vi "Weather Station UI.vi"(10 "Lower Limit":dbl=10.0, 11 "Upper Limit":dbl=30.0) -> (1 "Warning":string, 2 "Temperature History":dbl(graph))   [LabVIEW 2010]
doc: "This is the main VI in the Weather Station Project. It contains the user interface for a temperature warning system. \n\nUser inputs: Maximum Temperature, Minimum Temperature, Temperature Units.\nOutputs: Current Temperature, Warning State"
uses:
  Supporting Files/Weather Station States.ctl
panel:
  in  "Weather Data":dynamicdata(graph)
  in  "stop":bool
  in  "Wind Upper Limit":dbl(slide)=50.0 scale=0.0..100.0
  out "Wind Speed History":dbl(graph)
  # "Celcius"
  # "Temperature Ranges"
  # "Heat \nStroke"
  # "Freeze"
  # "kph"
  # "Maximum Safe Wind Speed"
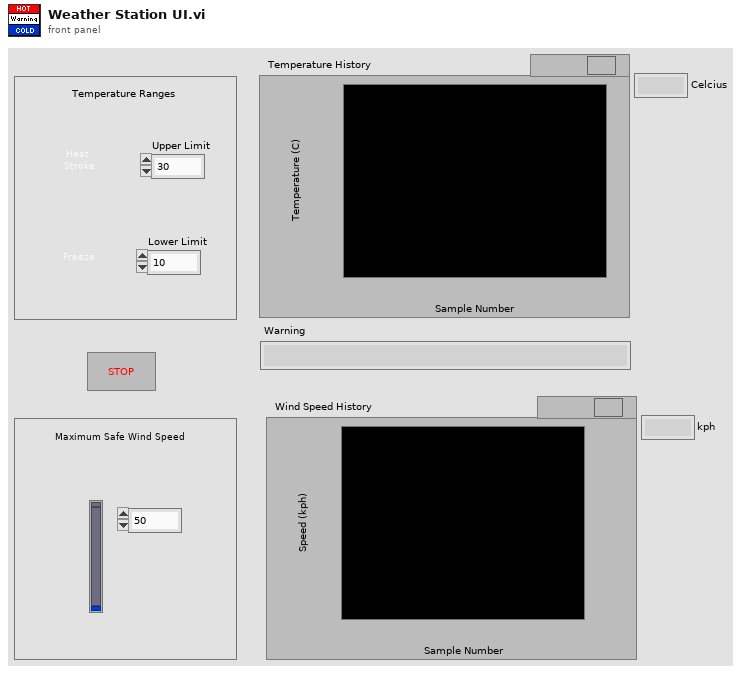
[diagram p1: front panel]
types:
  T1 = cluster{"Temperature":dbl, "T Upper Limit":dbl, "T Lower Limit":dbl, "Wind Speed":dbl, "Wind Upper Limit":dbl, "Warning":string, "Time":dbl}
  T2 = typedef "Weather Station States.ctl" = enum16{"Analysis", "Process UI", "Set Warning", "Data Log", "Stop"}
  T3 = enum32{"invalid app kind", "Development System", "Run Time System", "Student Edition", "Embedded LabVIEW", "Evaluation", "Custom"}
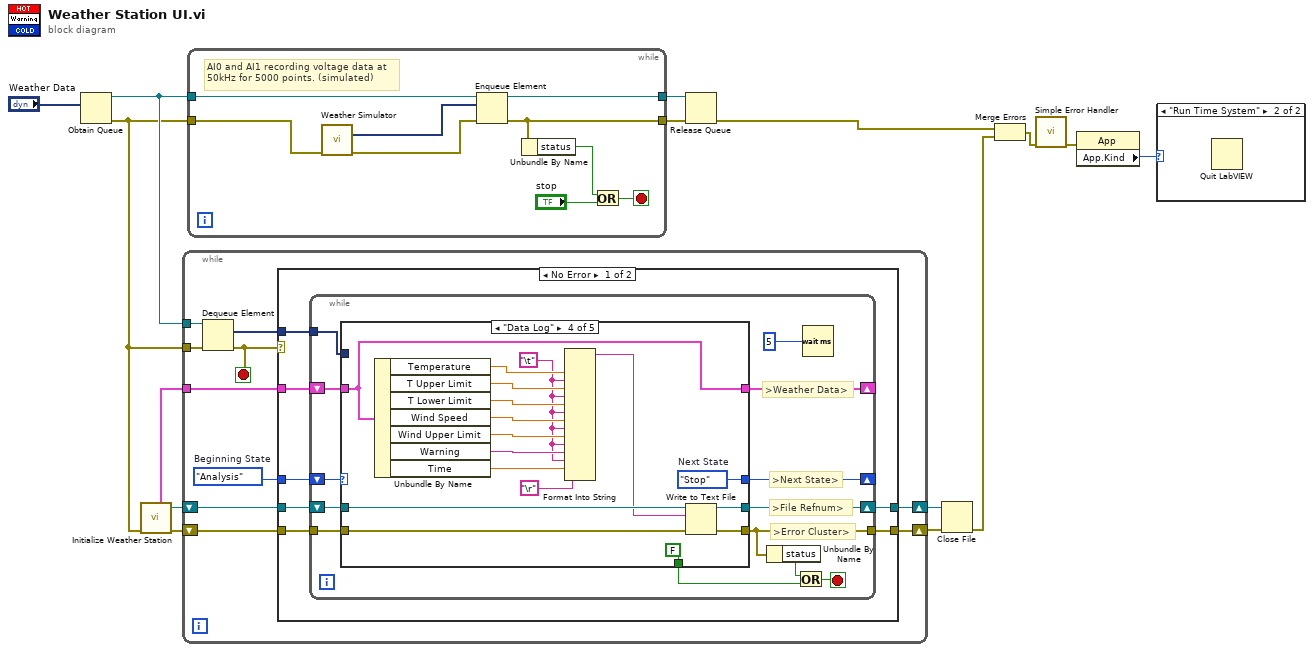
[diagram p0: block diagram]
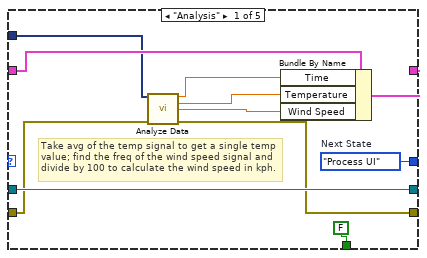
[diagram p3: hidden frame]
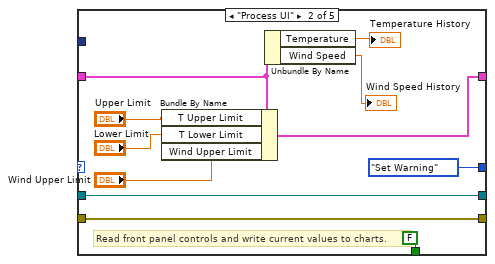
[diagram p4: hidden frame]
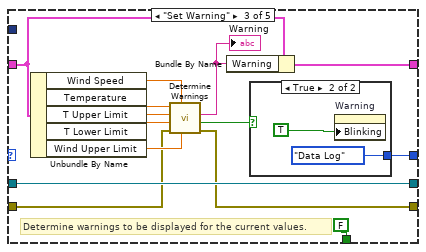
[diagram p5: hidden frame]
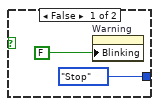
[diagram p6: hidden frame]
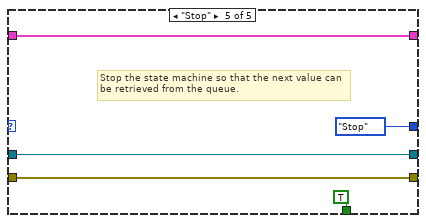
[diagram p7: hidden frame]
diagram:
  n1 = Obtain Queue(element data type="Weather Data") -> (queue out=w12:refnum<queue>, error out=w3:errorcluster)  [unwired: 4 in, 1 out]
  n2 = call "Initialize Weather Station.vi"("error in (no error)"=w3) -> ("error out"=w4:errorcluster, "file refnum"=w5:refnum<file>, "Weather Data"=w15:T1)  [unwired: 8 in]
  n3 = while {
    tunnel: w15 -> [w24]
    tunnel: w12 -> [w23]
    tunnel: w3 -> [w22]
    shift-right: [w25] -> w8
    shift-left: w5 -> [w21]
    shift-right: [w17] -> w7
    shift-left: w4 -> [w18]
    stop <- w20 stop-if-true
    w16 = Weather_Station_States."Analysis"  # Beginning State
    n4 = Dequeue Element(queue=w23, error in (no error)=w22) -> (element=w19:dynamicdata, error out=w20:errorcluster)  [unwired: 1 in, 2 out]
    n5 = case shown="No Error" w20 {
      tunnel: [w32 w108] -> w25
      tunnel: w24 -> [w31 _]
      tunnel: w21 -> [w30 w108]
      tunnel: w19 -> [w29 _]
      tunnel: w18 -> [w27 w109]
      tunnel: [w28 w109] -> w17
      tunnel: w16 -> [w26 _]
      frame No Error {
        n6 = while {
          shift-right: [w45] -> _
          shift-left: w26 -> [w37]
          shift-right: [w34] -> w32
          shift-left: w30 -> [w44]
          shift-right: [w38] -> _
          shift-left: w31 -> [w41]
          tunnel: w29 -> [w36]
          tunnel: [w35] -> w28
          tunnel: w27 -> [w33]
          stop <- w43 stop-if-true
          # ">Error Cluster>"
          # ">Weather Data>"
          # ">File Refnum>"
          # ">Next State>"
          n7 = case shown="\"Data Log\"" w37 {
            tunnel: [w56 Weather_Station_States."Set Warning" ("Next State") w80 w102 Weather_Station_States."Stop" ("Next State")] -> w45
            tunnel: [w46 w58 w70 w99 w103] -> w35
            tunnel: w44 -> [w52 w57 w77 w98 w104]
            tunnel: [w53 w67 w78 w96 w105] -> w38
            tunnel: w41 -> [w54 w64 w79 w96 w105]
            tunnel: [FALSE ("stop") FALSE ("stop") FALSE ("stop") FALSE ("stop") TRUE ("stop")] -> w40
            tunnel: w36 -> [w51 _ _ _ _]
            tunnel: [w52 w57 w77 w100 w104] -> w34
            tunnel: w33 -> [w50 w58 w71 w86 w103]
            frame "Analysis" {
              w56 = Weather_Station_States."Process UI"  # Next State
              # "Take avg of the temp signal to get a single temp value; find the freq of the wind speed signal and divide by 100 to calculate the wind speed in kph."
              n8 = call "Analyze Data.vi"("Weather Data"=w51, "error in"=w50) -> ("Time"=w49:dbl, "Temperature"=w48:dbl, "Wind Speed"=w47:dbl, "error out"=w46:errorcluster)  [unwired: 10 in]
              n9 = Bundle By Name(cluster=w54, "Time"=w49, "Temperature"=w48, "Wind Speed"=w47) -> (w53:T1)
            }
            frame "Process UI" {
              # "Read front panel controls and write current values to charts."
              n10 = Bundle By Name(cluster=w64, "T Upper Limit"="Upper Limit", "T Lower Limit"="Lower Limit", "Wind Upper Limit"="Wind Upper Limit") -> (w67:T1)
              n11 = Unbundle By Name(w64) -> ("Temperature"=→"Temperature History":dbl, "Wind Speed"=→"Wind Speed History":dbl)
            }
            frame "Set Warning" {
              # "Determine warnings to be displayed for the current values."
              n12 = Unbundle By Name(w79) -> ("Wind Speed"=w76:dbl, "Temperature"=w75:dbl, "T Upper Limit"=w74:dbl, "T Lower Limit"=w73:dbl, "Wind Upper Limit"=w72:dbl)
              n13 = call "Determine Warnings.vi"("Max Wind Speed"=w72, "Current Wind Speed"=w76, "error in (no error)"=w71, "Min Temp"=w73, "Max Temp"=w74, "Current Temp"=w75) -> ("error out"=w70:errorcluster, "Warning?"=w69:bool, "Warning Text"=w68:string)  [unwired: 3 in]
              "Warning" <- w68
              n14 = Bundle By Name(cluster=w79, "Warning"=w68) -> (w78:T1)
              n15 = case shown="True" w69 {
                tunnel: [Weather_Station_States."Stop" ("Next State") Weather_Station_States."Data Log" ("Next State")] -> w80
                frame False {
                  n16 = property on="Warning" class="Str"("Blinking"=FALSE) -> ()  [unwired: 2 in, 2 out]
                }
                frame True {
                  n17 = property on="Warning" class="Str"("Blinking"=TRUE) -> ()  [unwired: 2 in, 2 out]
                }
              }
            }
            frame "Data Log" {
              w88 = "\t"
              w102 = Weather_Station_States."Stop"  # Next State
              n18 = Unbundle By Name(w96) -> ("Temperature"=w95:dbl, "T Upper Limit"=w94:dbl, "T Lower Limit"=w93:dbl, "Wind Speed"=w92:dbl, "Wind Upper Limit"=w91:dbl, "Warning"=w90:string, "Time"=w89:dbl)
              n19 = Format Into String(w95, w88, w94, w88, w93, w88, w92, w88, w91, w88, w90, w88, w89, "\r") -> (resulting string=w97:string)  [unwired: 3 in, 1 out]
              n20 = Write to Text File(file (use dialog)=w98, text=w97, error in=w86) -> (refnum out=w100:refnum<file>, error out=w99:errorcluster)  [unwired: 1 in, 1 out]
            }
            frame "Stop" {
              # "Stop the state machine so that the next value can be retrieved from the queue."
            }
          }
          n21 = Unbundle By Name(w35) -> ("status"=w42:bool)
          n22 = Or(x=w42, y=w40) -> (x .or. y?=w43:bool)
          n23 = Wait (ms)(milliseconds to wait=u32 5 ("y")) -> ()  [unwired: 1 out]
        }
      }
      frame Error {
      }
    }
  }
  n24 = while {
    tunnel: w12 -> [w118]
    tunnel: w3 -> [w112]
    tunnel: [w115] -> w14
    tunnel: [w117] -> w13
    stop <- w113 stop-if-true
    # "AI0 and AI1 recording voltage data at 50kHz for 5000 points. (simulated)"
    n25 = call "Weather Simulator.vi"("error in (no error)"=w112) -> ("Waveform Graph"=w110:dynamicdata, "error out"=w111:errorcluster)  [unwired: 13 in]
    n26 = Enqueue Element(queue=w118, element=w110, error in (no error)=w111) -> (queue out=w117:refnum<queue>, error out=w115:errorcluster)  [unwired: 1 in, 1 out]
    n27 = Unbundle By Name(w115) -> ("status"=w114:bool)
    n28 = Or(x=w114, y="stop") -> (x .or. y?=w113:bool)
  }
  n29 = Release Queue(queue=w13, error in (no error)=w14) -> (error out=w10:errorcluster)  [unwired: 1 in, 2 out]
  n30 = Close File(refnum=w8, error in=w7) -> (error out=w6:errorcluster)  [unwired: 1 out]
  n31 = Merge Errors(w10, w6) -> (w9:errorcluster)
  n32 = call <vilib>:"Simple Error Handler.vi"("error in (no error)"=w9) -> ("error out"=w1:errorcluster)  [unwired: 4 in, 4 out]
  n33 = property class="App"(error in=w1) -> ("App.Kind"=w2:T3)  [unwired: 1 in, 2 out]
  n34 = case shown="\"Run Time System\"" w2 {
    frame "invalid app kind", Default {
    }
    frame "Run Time System" {
      n35 = Quit LabVIEW() -> ()  [unwired: 1 in]
    }
  }
